vi "Q8381 Loss Max Min Change .vi"(2 "LOSS Measure?":bool, 3 "Received Y: min":dbl format="%.4e", 4 "Received Y: max":dbl format="%.4e") -> (0 "Y: min":dbl format="%.4e", 1 "Y: max":dbl format="%.4e")   [LabVIEW 2017]
doc: "Change Max and Min of Y-axis if \"Loss\" is measured. Otherwise, this vi just passes received values.\nDefault:\n LOSS Measure? : False"
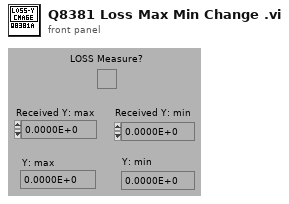
[diagram p1: front panel]
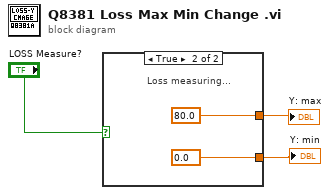
[diagram p0: block diagram]
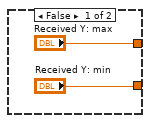
[diagram p2: hidden frame]
diagram:
  n1 = case shown="True" "LOSS Measure?" {
    tunnel: ["Received Y: max" 80.0] -> w2
    tunnel: ["Received Y: min" 0.0] -> w1
    frame False {
    }
    frame True {
      # "Loss measuring..."
    }
  }
  "Y: max" <- w2
  "Y: min" <- w1
